vi "Send Result to Python.vi"(5 "Error? (F)":bool, 6 "Python Message ID":i32, 7 "Server Alias":string, 8 "error in (no error)":errorcluster, 10 "Script ID":i64, 11 "Result Data":string[](array[string])) -> (0 "error out":errorcluster)   [LabVIEW 2013, in "TS.lvlib"]
doc: "If a Python script has asked LabVIEW to do something requiring a Result (the Reply is just an acknowledgement that LabVIEW got the message, but does not contain the Result), we send it back here. We have to keep track of the Script ID, since we could have multiple scripts running simultaneously."
uses:
  TS.lvlib
  LabVIEW Python Connector Message.ctl
panel:
  out "Message as sent":T1={"Command"="zxcvbnm,", "Data"=["asdfghjk", "qwertyui"], "Script ID"=0, "LabVIEW Server ID"="zxcvbnm,", "Python Message ID"=0}
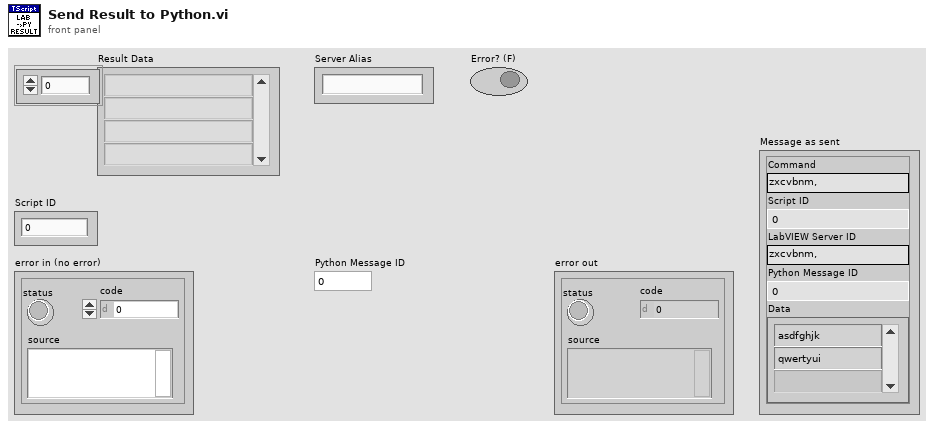
[diagram p1: front panel]
types:
  T1 = typedef "TS.lvlib/LabVIEW Python Connector Message.ctl" = cluster{"Command":string, "Data":string[], "Script ID":i64, "LabVIEW Server ID":string, "Python Message ID":i32}
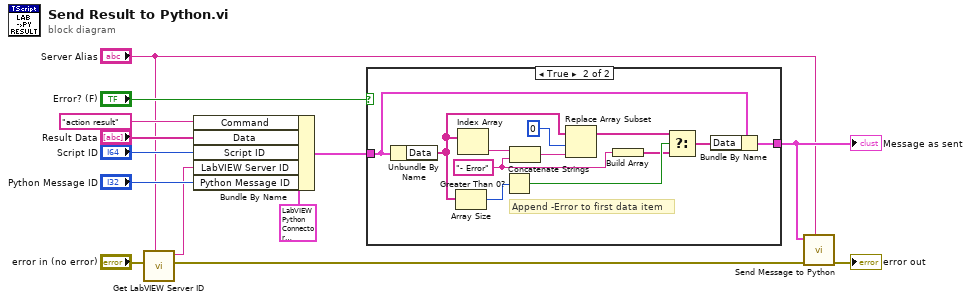
[diagram p0: block diagram]
diagram:
  n1 = call "Get LabVIEW Server ID.vi"("Server Alias"="Server Alias", "Error In"="error in (no error)") -> ("Error Out"=w3:errorcluster, "LabVIEW Server ID"=w1:string)  [unwired: 8 in]
  n2 = Bundle By Name(cluster=T1 {"Command"="xGetDMMVoltageReading", "Data"=["0.794077"], "Script ID"=0, "LabVIEW Server ID"="zxcvbnm,", "Python Message ID"=0} ("Message"), "Command"="action result" ("string"), "Data"="Result Data", "Script ID"="Script ID", "LabVIEW Server ID"=w1, "Python Message ID"="Python Message ID") -> (w12:T1)
  n3 = case shown="True" "Error? (F)" {
    tunnel: w12 -> [w14 w23]
    tunnel: [w14 w22] -> w9
    frame False {
    }
    frame True {
      w16 = "- Error" ("string")
      # "Append -Error to first data item"
      n4 = Unbundle By Name(w23) -> ("Data"=w21:string[])
      n5 = Array Size(array=w21) -> (size(s)=w20:i32)
      n6 = Index Array(array=w21) -> (element=w26:string)  [unwired: 1 in]
      n7 = Greater Than 0?(x=w20) -> (x > 0?=w19:bool)
      n8 = Concatenate Strings(w26, w16) -> (w25:string)
      n9 = Replace Array Subset(array=w21, new element=w25, index=0) -> (w18:string[])
      n10 = Build Array(w16) -> (w15:string[])
      n11 = Select(t=w18, s=w19, f=w15) -> (s? t:f=w17:string[])
      n12 = Bundle By Name(cluster=w23, "Data"=w17) -> (w22:T1)
    }
  }
  "Message as sent" <- w9
  n13 = call "Send Message to Python.vi"("Server Alias"="Server Alias", "error in (no error)"=w3, "Message"=w9) -> ("error out"=→"error out":errorcluster)  [unwired: 8 in]
